vi "Lookup Hardware by Name.vi"(8 "error in (no error)":errorcluster, 10 "Device Name":string, 11 "Controller in":refnum<class "Controller.lvclass">) -> (0 "error out":errorcluster, 2 "Hardware.lvclass":refnum<class "Hardware.lvclass">, 3 "Controller out":refnum<class "Controller.lvclass">)   [LabVIEW 2017, in "Controller Actor.lvlib" / "Controller.lvclass"]
uses:
  Controller.lvclass
  Hardware/Hardware.lvclass
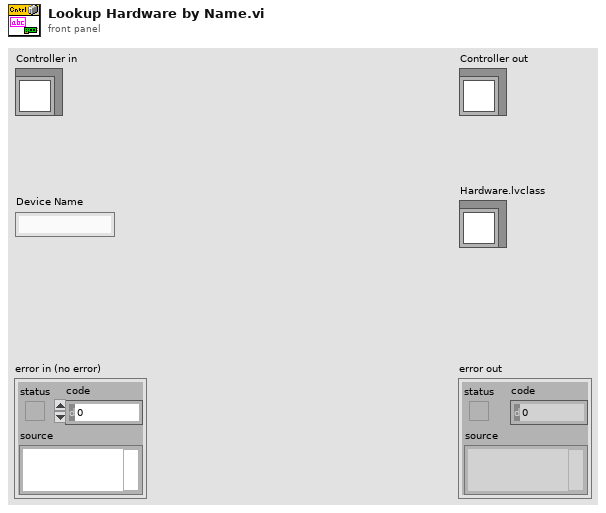
[diagram p1: front panel]
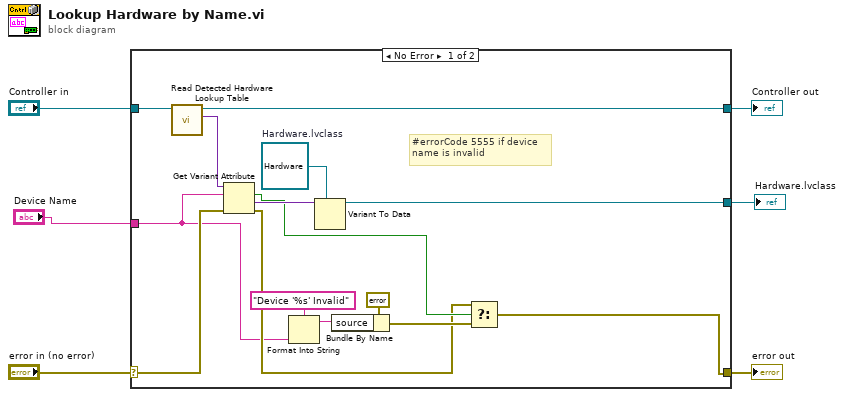
[diagram p0: block diagram]
diagram:
  n1 = case shown="No Error" "error in (no error)" {
    selector: "error in (no error)" -> [w15 w23]
    tunnel: [w7 w23] -> w5
    tunnel: [w20 w22] -> w3
    tunnel: "Controller in" -> [w21 w22]
    tunnel: "Device Name" -> [w8 _]
    tunnel: [w16 _] -> w1
    frame No Error {
      w19 = refnum<class "Hardware.lvclass"> refnum  # Hardware.lvclass
      # "#errorCode 5555 if device\nname is invalid"
      n2 = call "Read Detected Hardware Lookup Table.vi"("Controller in"=w21) -> ("Detected Hardware Lookup Table"=w18:variant, "Controller out"=w20:refnum<class "Controller.lvclass">)  [unwired: 8 in, 1 out]
      n3 = Get Variant Attribute(Variant=w18, name=w8, error in=w15) -> (found=w10:bool, value=w17:variant, error out=w9:errorcluster)  [unwired: 1 in, 1 out]
      n4 = Format Into String(format string="Device '%s' Invalid" ("source"), w8) -> (resulting string=w13:string)  [unwired: 2 in, 1 out]
      n5 = Variant To Data(type=w19, Variant=w17) -> (data=w16:refnum<class "Hardware.lvclass">)  [unwired: 1 in, 1 out]
      n6 = Bundle By Name(cluster=errorcluster {"status"=TRUE, "code"=5555, "source"="Device '%s' Invalid"} ("error constant"), "source"=w13) -> (w11:errorcluster)
      n7 = Select(t=w9, s=w10, f=w11) -> (s? t:f=w7:errorcluster)
    }
    frame Error {
    }
  }
  "error out" <- w5
  "Controller out" <- w3
  "Hardware.lvclass" <- w1
